vi "Parallel Loops.vi"() -> ()   [LabVIEW 2016]
uses:
  <vilib>/measure/madcrms.llb/Averaged DC-RMS for N Chan.vi
  <vilib>/measure/NI_MAPro.lvlib
panel:
  out "Bez DC":dynamicdata(graph)
  out "Acc 3 - Z":dbl
  out "Acc 3 - Y":dbl
  out "Acc 3 - X":dbl
  out "Acc 2 - Z":dbl
  out "Acc 2 - Y":dbl
  out "Acc 2 - X":dbl
  out "Acc 1 - Z":dbl
  out "Acc 1 - Y":dbl
  out "Acc 1 - X":dbl
  in  "DC vrednosti":bool
  out "Sekvenca":dbl[](array[numeric])
  out "Iter Score":i32
  out "Ulaz":dynamicdata(graph)
  out "#  in queue":i32
  out "Iter Akvizicija":i32
  in  "Treshold":dbl=1.0999999999999999 min=0.0 max=5.0 step=0.1
  out "Akvizicija":bool
  in  "Akvizicija - Start/Stop":string="N/A"
  out "Iter Sekvenca":i32
  in  "stop":bool
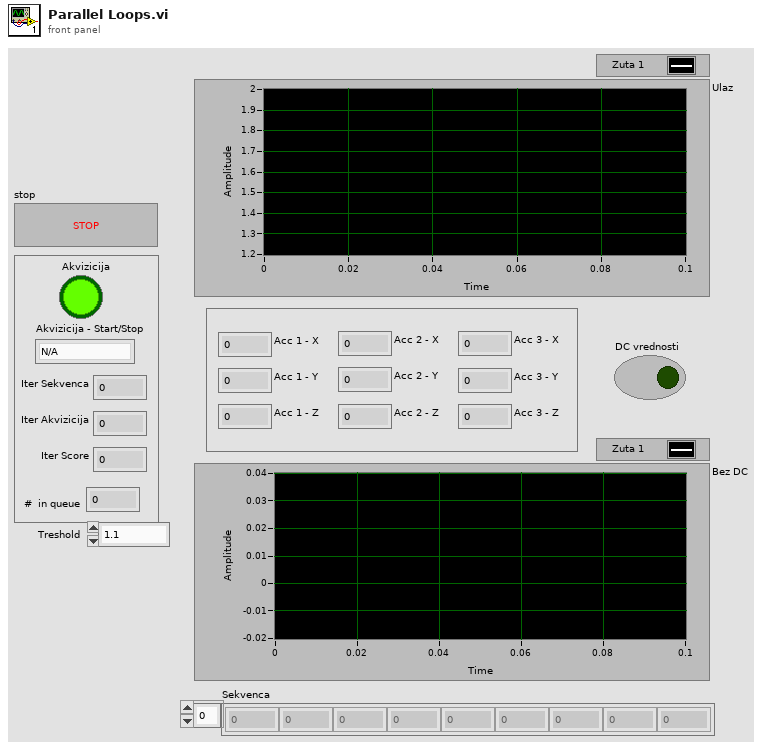
[diagram p1: front panel]
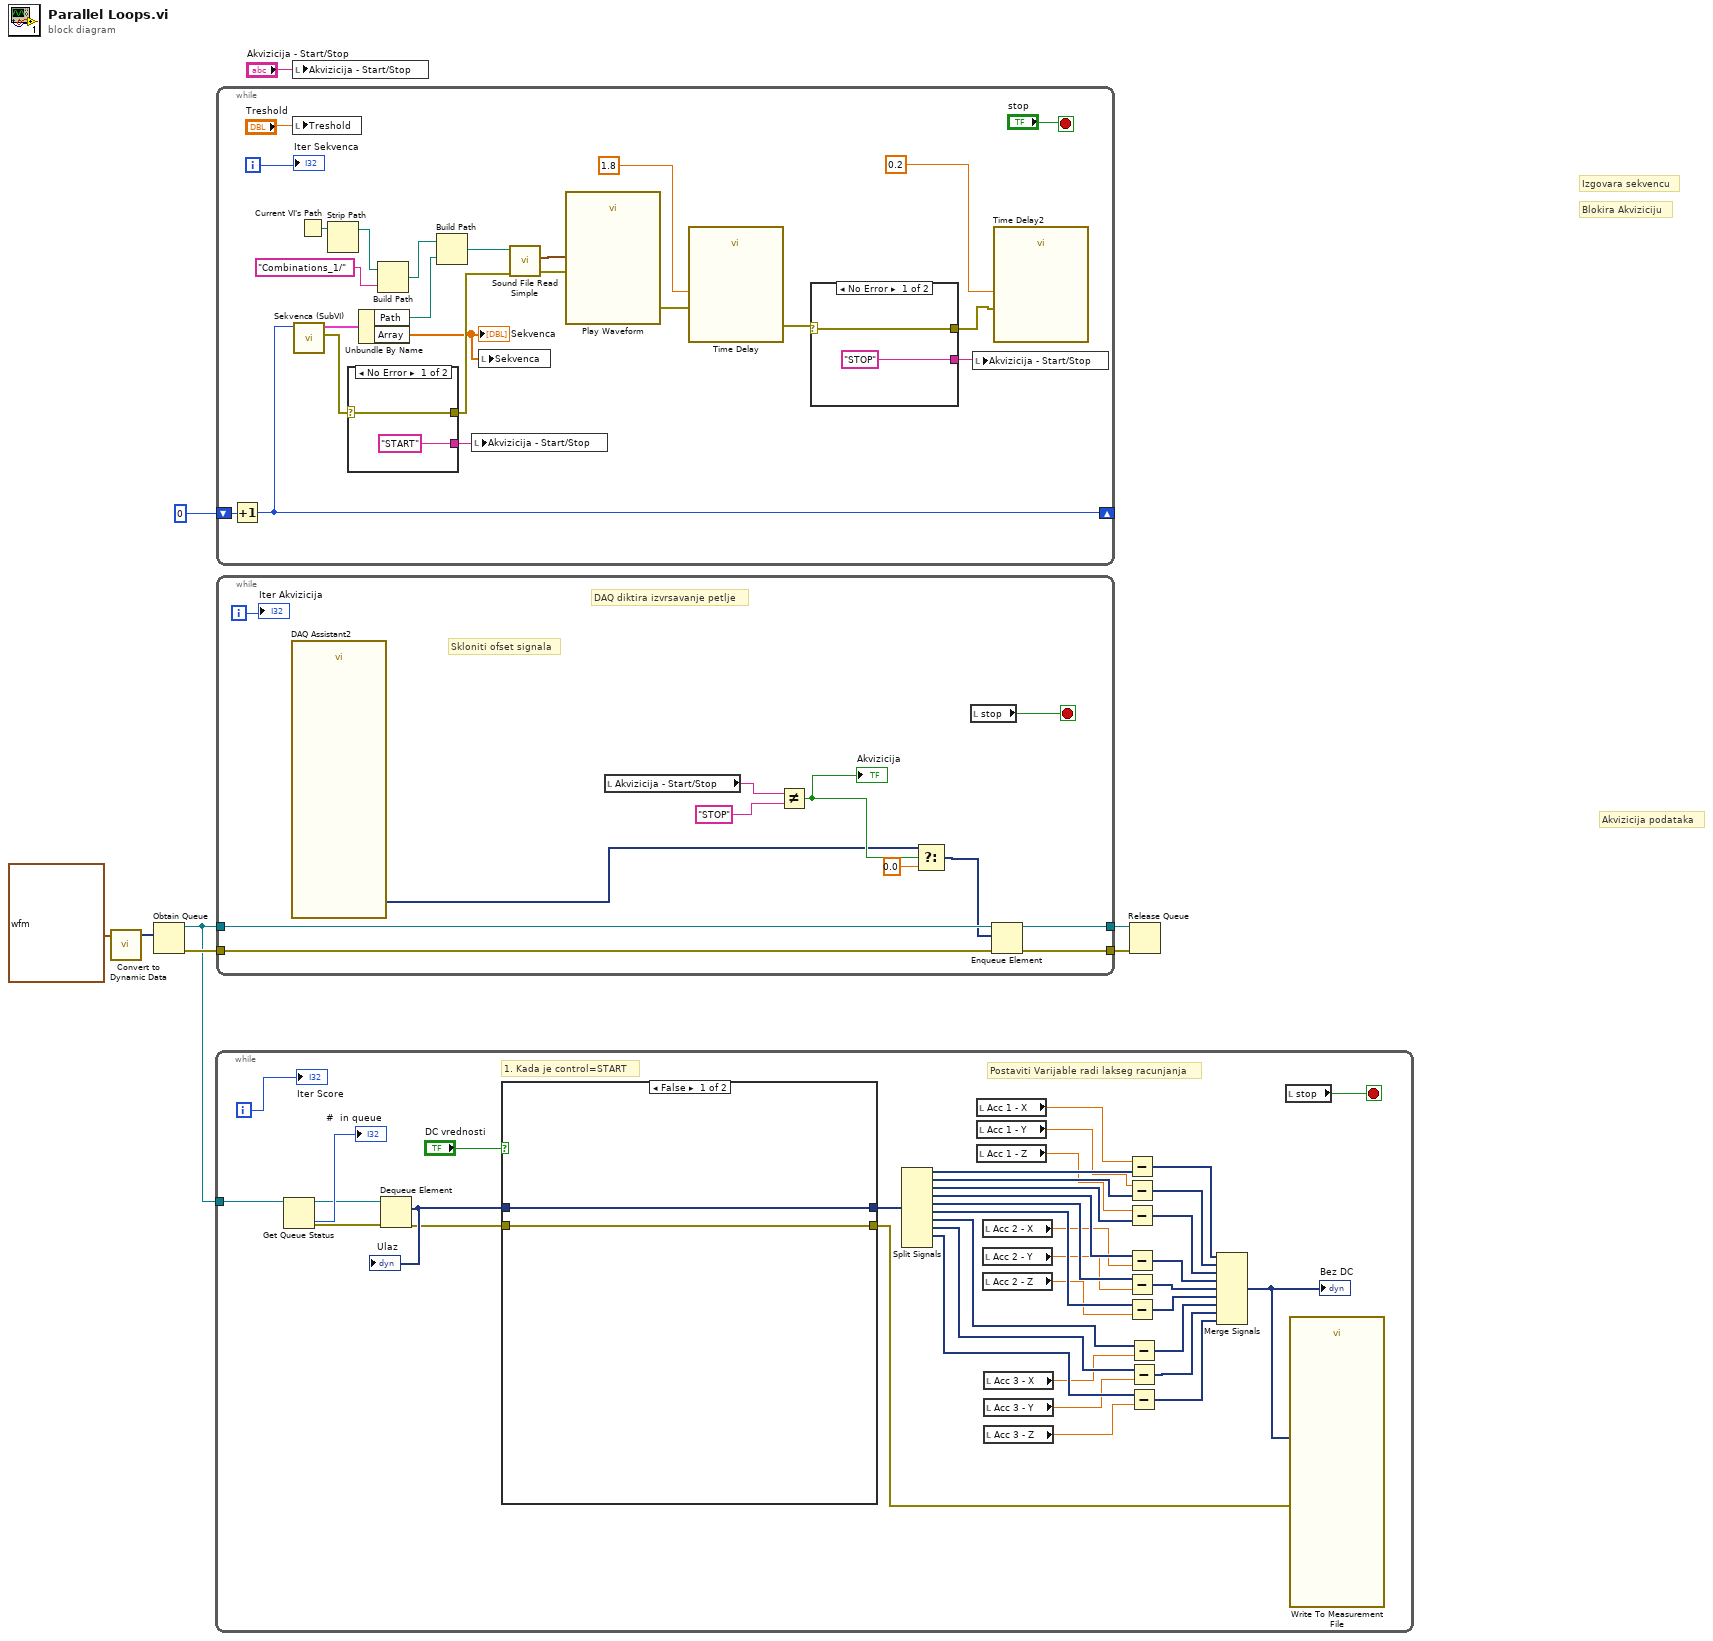
[diagram p0: block diagram]
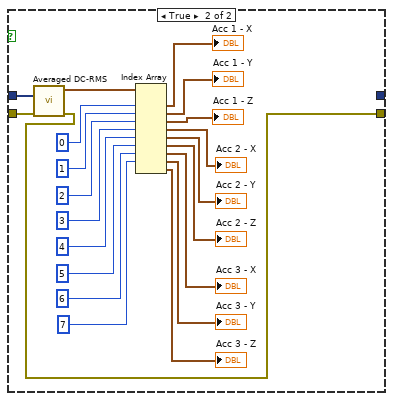
[diagram p2: hidden frame]
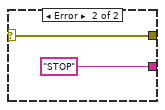
[diagram p3: hidden frame]
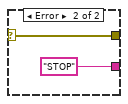
[diagram p4: hidden frame]
diagram:
  # "Akvizicija podataka"
  # "Blokira Akviziciju"
  # "Izgovara sekvencu"
  n1 = call "Convert to Dynamic Data"("Waveform"=waveform(dbl) {"t0"=timestamp(0 s since 1904-01-01), "dt"=1.0, "Y"=[]}) -> ("Dynamic Data Type"=w1:dynamicdata)  [unwired: 3 in]
  n2 = Obtain Queue(element data type=w1) -> (queue out=w3:refnum<queue>, error out=w6:errorcluster)  [unwired: 4 in, 1 out]
  n3 = while {
    tunnel: w3 -> [w46]
    i -> [w42]
    stop <- w47 stop-if-true
    # "Postaviti Varijable radi lakseg racunjanja"
    # "1. Kada je control=START"
    n4 = Get Queue Status(queue=w46) -> (queue out=w44:refnum<queue>, error out=w43:errorcluster, # elements in queue=→"#  in queue":i32)  [unwired: 2 in, 5 out]
    n5 = Dequeue Element(queue=w44, error in (no error)=w43) -> (element=w41:dynamicdata, error out=w11:errorcluster)  [unwired: 1 in, 2 out]
    "Ulaz" <- w41
    n6 = case shown="False" "DC vrednosti" {
      tunnel: w41 -> [w49 w70]
      tunnel: w11 -> [w48 w69]
      tunnel: [w49 _] -> w39
      tunnel: [w48 w51] -> w10
      frame False {
      }
      frame True {
        n7 = call-poly <vilib>:"Averaged DC-RMS.vi"("error in (no error)"=w69, "signals in"=w70) -> ("error out"=w51:errorcluster, "DC value waveforms"=w68:waveform(dbl)[])  [unwired: 5 in, 3 out]
        n8 = Index Array(array=w68, index #1=0, index #2=1, index #3=2, index #4=3, index #5=4, index #6=5, index #7=6, index #8=7) -> (element #1=→"Acc 1 - X":waveform(dbl), element #2=→"Acc 1 - Y":waveform(dbl), element #3=→"Acc 1 - Z":waveform(dbl), element #4=→"Acc 2 - X":waveform(dbl), element #5=→"Acc 2 - Y":waveform(dbl), element #6=→"Acc 2 - Z":waveform(dbl), element #7=→"Acc 3 - X":waveform(dbl), element #8=→"Acc 3 - Y":waveform(dbl), element #9=→"Acc 3 - Z":waveform(dbl))  [unwired: 1 in]
      }
    }
    n9 = Split Signals(w39) -> (w38:dynamicdata, w37:dynamicdata, w36:dynamicdata, w35:dynamicdata, w34:dynamicdata, w33:dynamicdata, w26:dynamicdata, w25:dynamicdata, w24:dynamicdata)  [unwired: 10 in, 1 out]
    n10 = local read "Acc 1 - X"() -> (w32:dbl)
    n11 = local read "Acc 1 - Y"() -> (w31:dbl)
    n12 = local read "Acc 1 - Z"() -> (w30:dbl)
    n13 = local read "Acc 2 - X"() -> (w29:dbl)
    n14 = local read "Acc 2 - Y"() -> (w28:dbl)
    n15 = local read "Acc 2 - Z"() -> (w27:dbl)
    n16 = local read "Acc 3 - X"() -> (w23:dbl)
    n17 = local read "Acc 3 - Y"() -> (w22:dbl)
    n18 = local read "Acc 3 - Z"() -> (w21:dbl)
    n19 = Subtract(x=w32, y=w38) -> (x-y=w20:dynamicdata)
    n20 = Subtract(x=w31, y=w37) -> (x-y=w19:dynamicdata)
    n21 = Subtract(x=w30, y=w36) -> (x-y=w18:dynamicdata)
    n22 = Subtract(x=w35, y=w29) -> (x-y=w17:dynamicdata)
    n23 = Subtract(x=w34, y=w28) -> (x-y=w16:dynamicdata)
    n24 = Subtract(x=w33, y=w27) -> (x-y=w15:dynamicdata)
    n25 = Subtract(x=w26, y=w23) -> (x-y=w14:dynamicdata)
    n26 = Subtract(x=w25, y=w22) -> (x-y=w13:dynamicdata)
    n27 = Subtract(x=w24, y=w21) -> (x-y=w12:dynamicdata)
    n28 = Merge Signals(w20, w19, w18, w17, w16, w15, w14, w13, w12) -> (w9:dynamicdata)
    "Bez DC" <- w9
    n29 = local read "stop"() -> (w47:bool)
    n30 = call "Write To Measurement File"("Signals"=w9, "error in (no error)"=w10) -> ()  [unwired: 15 in, 3 out]
    "Iter Score" <- w42
  }
  n31 = while {
    shift-right: [w72] -> _
    shift-left: 0 -> [w84]
    i -> [w83]
    stop <- "stop" stop-if-true
    n32 = Increment(x=w84) -> (x+1=w72:i32)
    n33 = local write "Treshold"("Treshold") -> ()
    n34 = call "Sekvenca (SubVI).vi"("Ulaz"=w72) -> ("error out"=w82:errorcluster, "Cluster 41"=w86:cluster{"Path":path, "Array":dbl[]})  [unwired: 9 in]
    n35 = Current VI's Path() -> (path=w93:path)
    n36 = Strip Path(path=w93) -> (stripped path=w90:path)  [unwired: 1 out]
    n37 = case shown="No Error" w82 {
      selector: w82 -> [w99 w101]
      tunnel: ["START" "STOP"] -> w80
      tunnel: [w99 w101] -> w81
      frame No Error {
      }
      frame Error {
      }
    }
    n38 = Unbundle By Name(w86) -> ("Path"=w87:path, "Array"=w71:dbl[])
    "Sekvenca" <- w71
    n39 = Build Path(base path=w90, name or relative path="Combinations_1/") -> (appended path=w92:path)
    n40 = Build Path(base path=w92, name or relative path=w87) -> (appended path=w91:path)
    n41 = local write "Akvizicija - Start/Stop"(w80) -> ()
    n42 = local write "Sekvenca"(w71) -> ()
    n43 = call <vilib>:"Sound File Read Simple.vi"("error in (no error)"=w81, "path"=w91) -> ("error out"=w94:errorcluster, "data"=w88:waveform(dbl)[])  [unwired: 6 in, 2 out]
    n44 = call "Play Waveform"("Data"=w88, "error in"=w94) -> ("error out"=w78:errorcluster)  [unwired: 17 in]
    n45 = call "Time Delay"("error in (no error)"=w78, "Delay Time (s)"=1.8) -> ("error out"=w77:errorcluster)  [unwired: 9 in]
    n46 = case shown="No Error" w77 {
      selector: w77 -> [w95 w97]
      tunnel: ["STOP" "STOP"] -> w79
      tunnel: [w95 w97] -> w76
      frame No Error {
      }
      frame Error {
      }
    }
    n47 = local write "Akvizicija - Start/Stop"(w79) -> ()
    n48 = call "Time Delay2"("error in (no error)"=w76, "Delay Time (s)"=0.2) -> ()  [unwired: 9 in, 1 out]
    "Iter Sekvenca" <- w83
  }
  n49 = while {
    tunnel: w6 -> [w111]
    tunnel: w3 -> [w110]
    tunnel: [w108] -> w5
    tunnel: [w107] -> w4
    i -> [w112]
    stop <- w109 stop-if-true
    # "Skloniti ofset signala"
    # "DAQ diktira izvrsavanje petlje"
    n50 = call "DAQ Assistant2"() -> ("data"=w103:dynamicdata)  [unwired: 16 in, 3 out]
    n51 = local read "Akvizicija - Start/Stop"() -> (w113:string)
    n52 = Not Equal?(x=w113, y="STOP") -> (x != y?=w106:bool)
    "Akvizicija" <- w106
    n53 = Select(t=w103, s=w106, f=0.0) -> (s? t:f=w105:dynamicdata)
    n54 = local read "stop"() -> (w109:bool)
    n55 = Enqueue Element(queue=w110, element=w105, error in (no error)=w111) -> (queue out=w108:refnum<queue>, error out=w107:errorcluster)  [unwired: 1 in, 1 out]
    "Iter Akvizicija" <- w112
  }
  n56 = local write "Akvizicija - Start/Stop"("Akvizicija - Start/Stop") -> ()
  n57 = Release Queue(queue=w5, error in (no error)=w4) -> ()  [unwired: 1 in, 3 out]
